vi "Thorlabs Module.vi"(7 "Actions":T3(ring)=enum."Generate Scan Pattern", 8 "error in":errorcluster, 9 "Objective":u16(ring)=1 items=["5X LKM05", "10X LKM10", "20X LKM20", "10X LSM02"], 10 "ROI Parameters":T1={"ROI (mm)"={"X (mm)"=1.0, "Y (mm)"=1.0}, "Shift (mm)"={"Xshift (mm)"=0.0, "Yshift (mm)"=0.0}}, 11 "Scan Parameters":T2={"# Scan"={"#Ascan"=400, "#Bscan"=400}, "# Rpt"={"#ARpt"=1, "#BRpt"=1}, "Aline Rate"=2, "# Extra"={"# ARpt_extra"=5, "#Brtn_extra"=60}} {"Aline Rate" items=["76 KHz", "146 KHz", "76 KHz", "28 KHz", "10 KHz"]}) -> (0 "error out":errorcluster, 2 "Data Out":sgl[][](array[numeric]), 3 "Raw Data Out":u16[][](array[numeric]), 4 "#Blines":dbl)   [LabVIEW 2018]
uses:
  Hardware Mfg/Thorlabs OCT/SpectralRadar/LabVIEW/2012/user.lib/SpectralRadar.llb/Processing Flag Selection.ctl
  Hardware Mfg/Thorlabs OCT/SpectralRadar/LabVIEW/2012/user.lib/SpectralRadar.llb/Probe Parameter Int Selection.ctl
  Hardware Mfg/Thorlabs OCT/SpectralRadar/LabVIEW/2012/user.lib/SpectralRadar.llb/Scan Pattern.lvclass
  Hardware Mfg/Thorlabs OCT/SpectralRadar/LabVIEW/2012/user.lib/SpectralRadar.llb/set Spectrum Output.vi
  Hardware Mfg/Thorlabs OCT/SpectralRadar/LabVIEW/2012/user.lib/SpectralRadar.llb/set Scan Output.vi
  Hardware Mfg/Thorlabs OCT/SpectralRadar/LabVIEW/2012/user.lib/SpectralRadar.llb/Data.lvclass
  Hardware Mfg/Thorlabs OCT/SpectralRadar/LabVIEW/2012/user.lib/SpectralRadar.llb/Raw Data.lvclass
  Hardware Mfg/Thorlabs OCT/SpectralRadar/LabVIEW/2012/user.lib/SpectralRadar.llb/Processing.lvclass
  Hardware Mfg/Thorlabs OCT/SpectralRadar/LabVIEW/2012/user.lib/SpectralRadar.llb/Probe.lvclass
  Hardware Mfg/Thorlabs OCT/SpectralRadar/LabVIEW/2012/user.lib/SpectralRadar.llb/OCT Device.lvclass
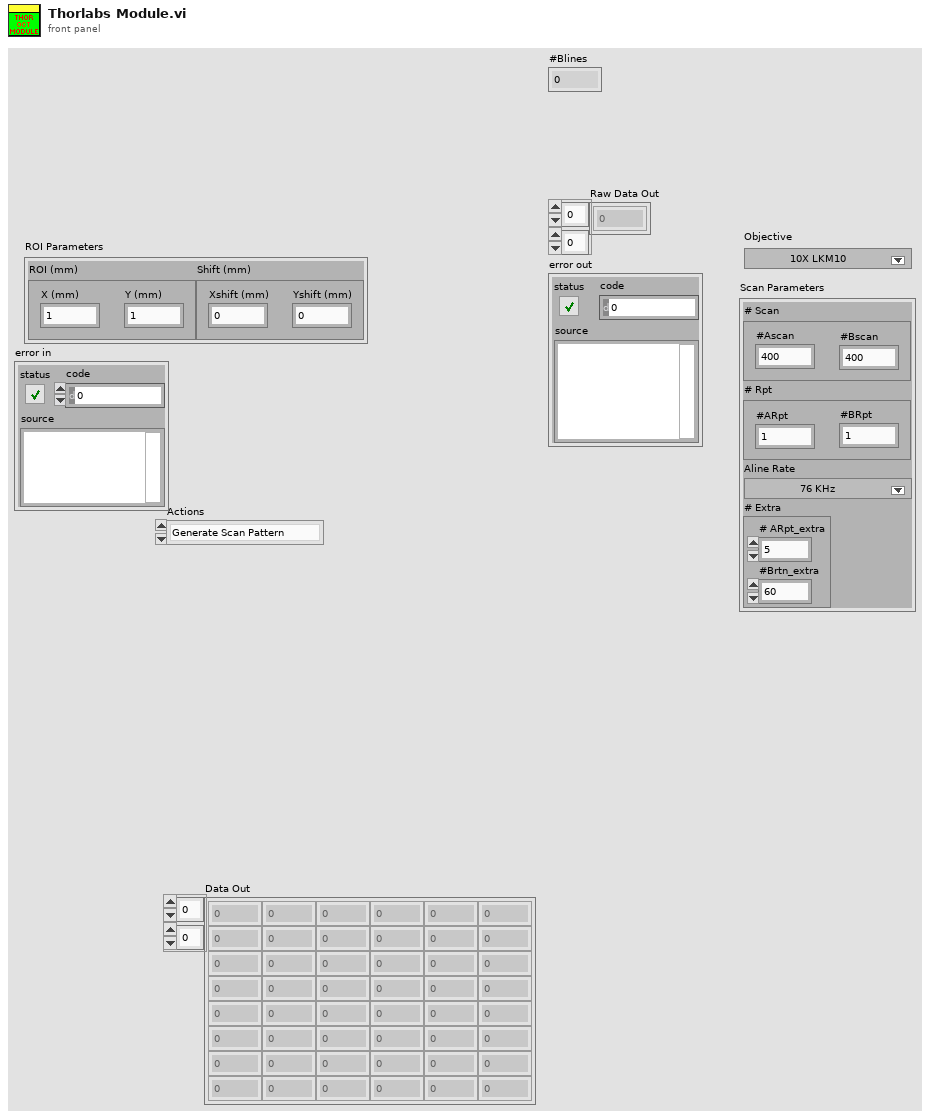
[diagram p1: front panel]
types:
  T1 = cluster{"ROI (mm)":cluster{"X (mm)":dbl, "Y (mm)":dbl}, "Shift (mm)":cluster{"Xshift (mm)":sgl, "Yshift (mm)":sgl}}
  T2 = cluster{"# Scan":cluster{"#Ascan":i32, "#Bscan":i32}, "# Rpt":cluster{"#ARpt":i32, "#BRpt":i32}, "Aline Rate":u16, "# Extra":cluster{"# ARpt_extra":i32, "#Brtn_extra":i32}}
  T3 = enum16{"Init", "Configure", "Configure Data", "Generate Scan Pattern", "Start Acquire Raw", "Start Acquire Data", "Acquire RAW", "Acquire Data", "Stop Acquire", "Uninit"}
  T4 = typedef "Processing.lvclass/Processing Flag Selection.ctl" = enum16{"Use Offset Errors", "Remove DC Spectrum", "Remove Advanced DC Spectrum", "Use Apodization", "Use Scan For Apodization", "Filter Undersampled Signals", "Use Dispersion Compensation", "Use Dechirp", "Use Extended Adjust", "Full Range Output", "Filter DC", "Autocorrelation Compensation", "DEFR", "Only Windowing", "Remove Fixed Pattern"}
  T5 = enum16{"FreeRunning", "TrigBoard_ExternalStart", "External_AScan"}
  T6 = typedef "Probe.lvclass/Probe Parameter Int Selection.ctl" = enum16{"Apodization Cycles", "Oversampling", "White Balance Auto", "Oversampling Slow Axis"}
  T7 = enum16{"Asynchronous Continuous", "Asynchronous Finite", "Synchronous"}
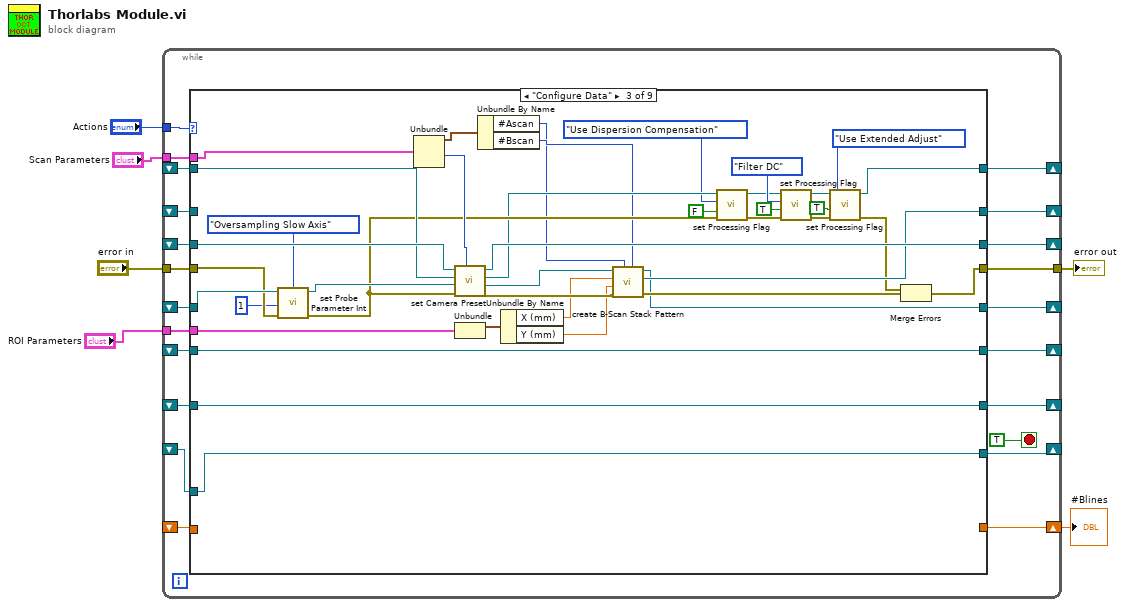
[diagram p0: block diagram]
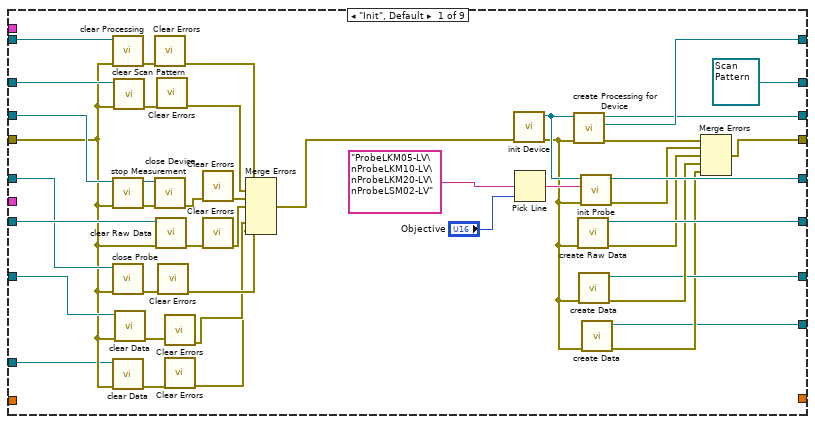
[diagram p2: hidden frame]
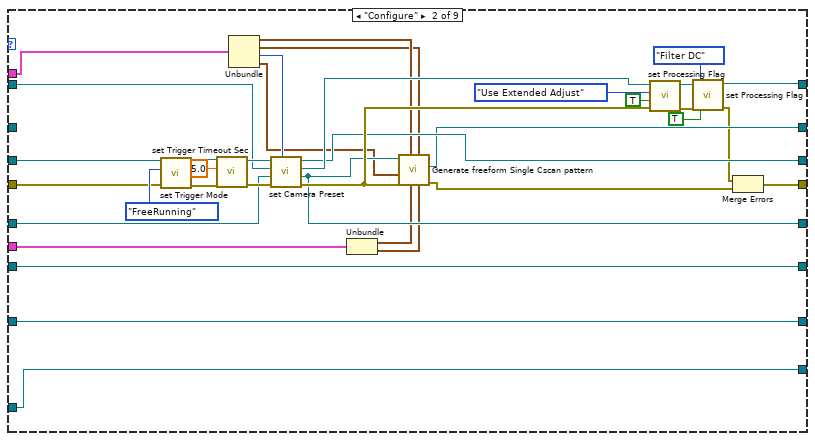
[diagram p3: hidden frame]
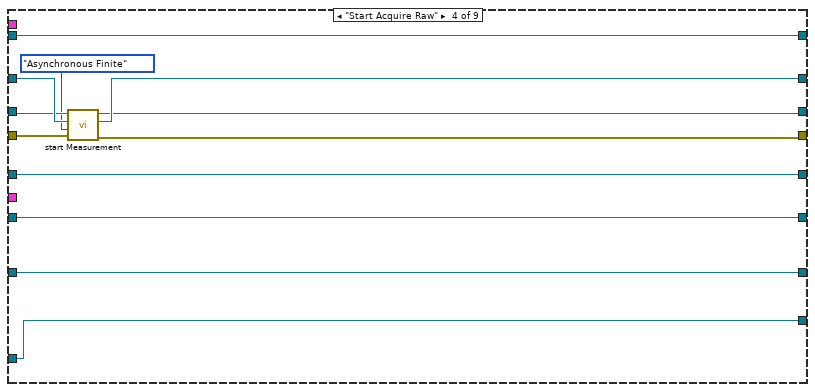
[diagram p4: hidden frame]
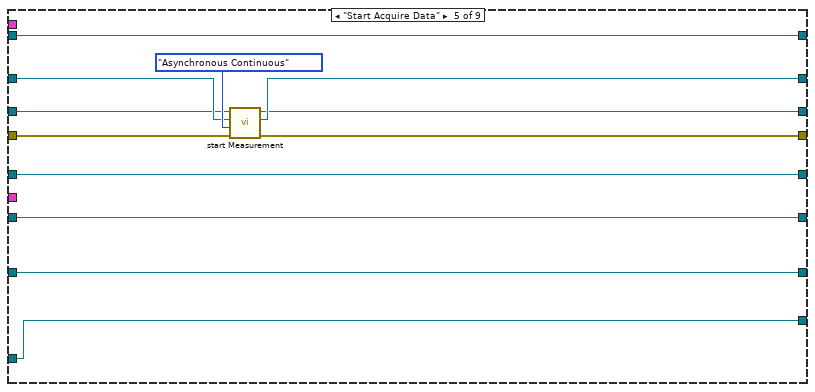
[diagram p5: hidden frame]
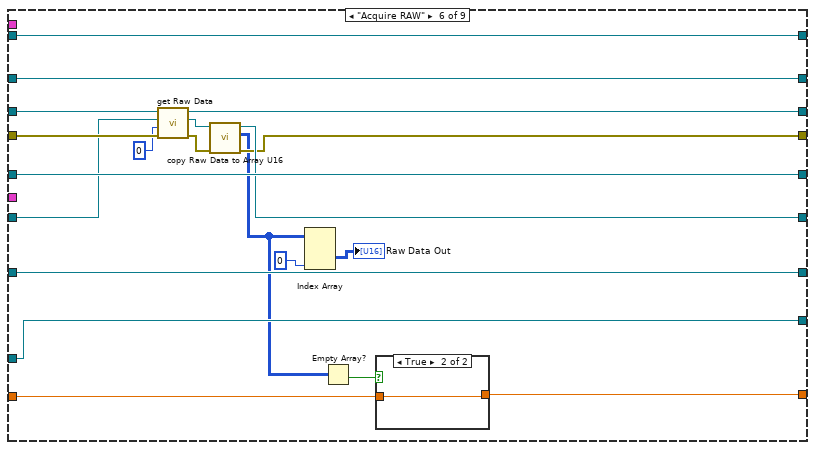
[diagram p6: hidden frame]
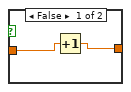
[diagram p7: hidden frame]
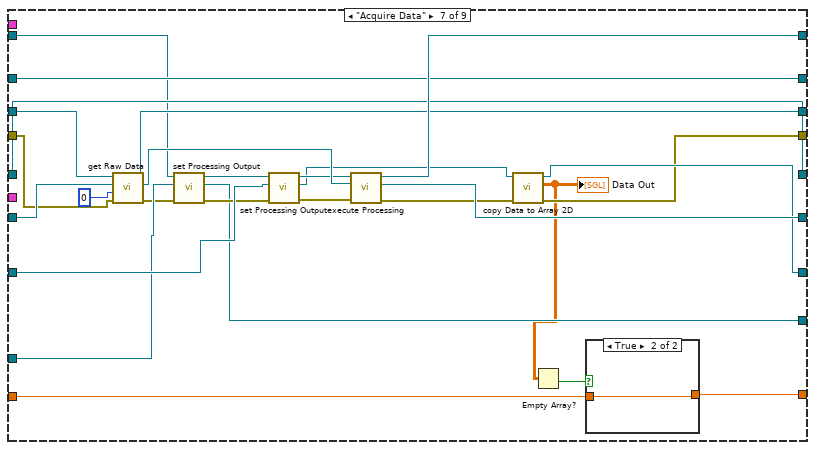
[diagram p8: hidden frame]
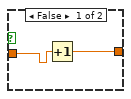
[diagram p9: hidden frame]
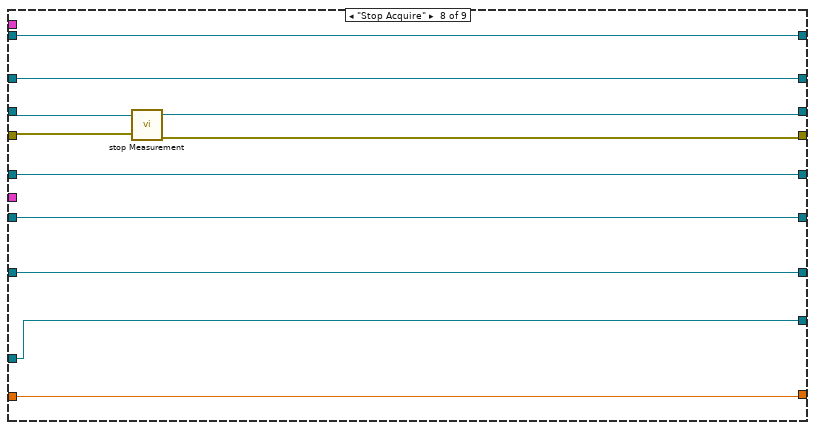
[diagram p10: hidden frame]
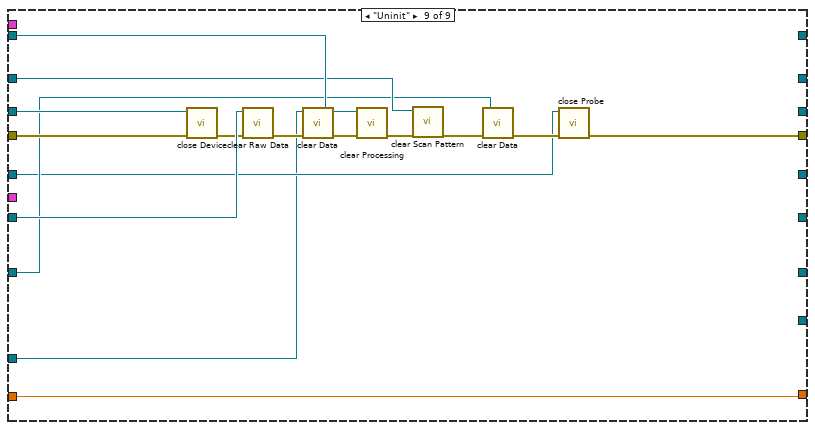
[diagram p11: hidden frame]
diagram:
  n1 = while {
    tunnel: "Actions" -> [w28]
    shift-right: [w26] -> _
    shift-left: _ -> [w22]
    shift-right: [w23] -> _
    shift-left: _ -> [w21]
    shift-right: [w20] -> _
    shift-left: _ -> [w19]
    shift-right: [w18] -> _
    shift-left: _ -> [w17]
    shift-right: [w16] -> _
    shift-left: _ -> [w15]
    tunnel: "error in" -> [w24]
    tunnel: [w25] -> w5
    shift-right: [w14] -> _
    shift-left: _ -> [w13]
    shift-right: [w12] -> _
    shift-left: _ -> [w11]
    tunnel: "Scan Parameters" -> [w10]
    tunnel: "ROI Parameters" -> [w9]
    shift-right: [w8] -> w1
    shift-left: _ -> [w7]
    stop <- TRUE stop-if-true
    n2 = case shown="\"Configure Data\"" w28 {
      tunnel: [w58 w94 w143 w154 w165 w185 w213 w232 _] -> w26
      tunnel: [w64 w106 w132 w158 w169 w180 w199 w234 w241] -> w25
      tunnel: w24 -> [w33 w84 w140 w159 w170 w189 w212 w235 w245]
      tunnel: [w66 w95 w127 w152 w163 w190 w215 w229 _] -> w23
      tunnel: w22 -> [w55 w83 w144 w155 w166 w187 w220 w233 w249]
      tunnel: w21 -> [w52 w78 w142 w152 w163 w190 w215 w229 w240]
      tunnel: [w60 w74 w111 w153 w164 w191 w217 w230 _] -> w20
      tunnel: w19 -> [w50 w85 w137 w153 w164 w191 w209 w230 w248]
      tunnel: [w67 w97 w130 w151 w162 w181 w214 w228 _] -> w18
      tunnel: w17 -> [w53 w97 w130 w151 w162 w186 w221 w228 w251]
      tunnel: [refnum<class "Scan Pattern.lvclass"> refnum ("Scan Pattern") w93 w131 w156 w167 w184 w216 w231 _] -> w16
      tunnel: w15 -> [w51 _ _ w157 w168 w184 w216 w231 w246]
      tunnel: [w45 w82 w129 w149 w161 w177 w202 w227 _] -> w14
      tunnel: w13 -> [w43 w82 w129 w149 w161 w177 w211 w227 w244]
      tunnel: [w34 w81 w128 w148 w160 w176 w201 w226 _] -> w12
      tunnel: w11 -> [w30 w81 w128 w148 w160 w176 w210 w226 w237]
      tunnel: w10 -> [_ w80 w126 _ _ _ _ _ _]
      tunnel: w9 -> [_ w79 w125 _ _ _ _ _ _]
      tunnel: w7 -> [_ _ _ _ _ w173 w196 w225 w236]
      tunnel: [_ _ _ _ _ w172 w195 w225 w236] -> w8
      frame "Init", Default {
        n3 = call "clear Processing.vi"("error in (no error)"=w33, "Processing"=w50) -> ("error out"=w49:errorcluster)  [unwired: 5 in]
        n4 = call "stop Measurement.vi"("error in (no error)"=w33, "OCTDevice"=w55) -> ("error out"=w57:errorcluster, "OCTDevice"=w56:refnum<class "OCT Device.lvclass">)  [unwired: 4 in]
        n5 = call "close Probe.vi"("error in (no error)"=w33, "GalvoControl"=w52) -> ("error out"=w48:errorcluster)  [unwired: 5 in]
        n6 = call "clear Data.vi"("error in (no error)"=w33, "Data"=w30) -> ("error out"=w32:errorcluster)  [unwired: 5 in]
        n7 = call "clear Scan Pattern.vi"("error in (no error)"=w33, "Scan Pattern in"=w51) -> ("error out"=w47:errorcluster)  [unwired: 5 in]
        n8 = call "clear Data.vi"("error in (no error)"=w33, "Data"=w43) -> ("error out"=w44:errorcluster)  [unwired: 5 in]
        n9 = call <vilib>:"Clear Errors.vi"("error in (no error)"=w49) -> ("error out"=w42:errorcluster)  [unwired: 5 in, 1 out]
        n10 = call "close Device.vi"("error in (no error)"=w57, "OCTDevice"=w56) -> ("error out"=w69:errorcluster)  [unwired: 5 in]
        n11 = call "clear Raw Data.vi"("error in (no error)"=w33, "Raw Data"=w53) -> ("error out"=w68:errorcluster)  [unwired: 5 in]
        n12 = call <vilib>:"Clear Errors.vi"("error in (no error)"=w47) -> ("error out"=w41:errorcluster)  [unwired: 5 in, 1 out]
        n13 = call <vilib>:"Clear Errors.vi"("error in (no error)"=w48) -> ("error out"=w38:errorcluster)  [unwired: 5 in, 1 out]
        n14 = call <vilib>:"Clear Errors.vi"("error in (no error)"=w44) -> ("error out"=w37:errorcluster)  [unwired: 5 in, 1 out]
        n15 = call <vilib>:"Clear Errors.vi"("error in (no error)"=w32) -> ("error out"=w31:errorcluster)  [unwired: 5 in, 1 out]
        n16 = call <vilib>:"Clear Errors.vi"("error in (no error)"=w69) -> ("error out"=w40:errorcluster)  [unwired: 5 in, 1 out]
        n17 = call <vilib>:"Clear Errors.vi"("error in (no error)"=w68) -> ("error out"=w39:errorcluster)  [unwired: 5 in, 1 out]
        n18 = Merge Errors(w42, w41, w40, w39, w38, w37, w31) -> (w35:errorcluster)
        n19 = call "init Device.vi"("error in (no error)"=w35) -> ("error out"=w29:errorcluster, "OCTDevice"=w61:refnum<class "OCT Device.lvclass">)  [unwired: 5 in]
        n20 = Pick Line(multi-line string="ProbeLKM05-LV\nProbeLKM10-LV\nProbeLKM20-LV\nProbeLSM02-LV" ("string (\"\")"), line index="Objective") -> (output string=w65:string)  [unwired: 1 in]
        n21 = call "create Processing for Device.vi"("error in (no error)"=w29, "OCTDevice"=w61) -> ("error out"=w59:errorcluster, "Processing"=w60:refnum<class "Processing.lvclass">, "OCTDevice"=w58:refnum<class "OCT Device.lvclass">)  [unwired: 3 in]
        n22 = call "create Raw Data.vi"("error in (no error)"=w29) -> ("error out"=w62:errorcluster, "Raw Data"=w67:refnum<class "Raw Data.lvclass">)  [unwired: 5 in]
        n23 = call "create Data.vi"("error in (no error)"=w29) -> ("error out"=w46:errorcluster, "Data"=w45:refnum<class "Data.lvclass">)  [unwired: 5 in]
        n24 = call "init Probe.vi"("error in (no error)"=w29, "Probe"=w65, "OCT Device"=w61) -> ("error out"=w63:errorcluster, "GalvoControl"=w66:refnum<class "Probe.lvclass">)  [unwired: 3 in]
        n25 = call "create Data.vi"("error in (no error)"=w29) -> ("error out"=w36:errorcluster, "Data"=w34:refnum<class "Data.lvclass">)  [unwired: 5 in]
        n26 = Merge Errors(w59, w63, w62, w46, w36) -> (w64:errorcluster)
      }
      frame "Configure" {
        n27 = call "set Trigger Mode.vi"("error in (no error)"=w84, "Trigger Type"=T5."FreeRunning", "OCTDevice in"=w83) -> ("error out"=w105:errorcluster, "OCTDevice out"=w107:refnum<class "OCT Device.lvclass">)  [unwired: 3 in]
        n28 = call "set Trigger Timeout Sec.vi"("error in (no error)"=w105, "Trigger Timeout"=5.0, "OCTDevice in"=w107) -> ("error out"=w99:errorcluster, "OCTDevice out"=w98:refnum<class "OCT Device.lvclass">)  [unwired: 3 in]
        n29 = Unbundle(w80) -> ("# Scan"=w90:cluster{"#Ascan":i32, "#Bscan":i32}, "# Rpt"=w89:cluster{"#ARpt":i32, "#BRpt":i32}, "Aline Rate"=w91:u16, "# Extra"=w86:cluster{"# ARpt_extra":i32, "#Brtn_extra":i32})
        n30 = call "set Camera Preset.vi"("Numeric"=w91, "error in (no error)"=w99, "Probe"=w78, "Processing"=w85, "OCTDevice"=w98) -> ("error out"=w96:errorcluster, "Probe 2"=w95:refnum<class "Probe.lvclass">, "Processing"=w100:refnum<class "Processing.lvclass">, "OCTDevice out"=w94:refnum<class "OCT Device.lvclass">)  [unwired: 1 in]
        n31 = Unbundle(w79) -> ("ROI (mm)"=w88:cluster{"X (mm)":dbl, "Y (mm)":dbl}, "Shift (mm)"=w87:cluster{"Xshift (mm)":sgl, "Yshift (mm)":sgl})
        n32 = call "Generate freeform Single Cscan pattern.vi"("Shift (mm)"=w87, "# Rpt"=w89, "ROI (mm)"=w88, "# Scan"=w90, "error in (no error)"=w96, "# Extra"=w86, "Probe"=w95) -> ("error out"=w92:errorcluster, "Scan Pattern"=w93:refnum<class "Scan Pattern.lvclass">)  [unwired: 1 in, 2 out]
        n33 = call "set Processing Flag.vi"("error in (no error)"=w96, "Flag"=TRUE, "Processing Flag Selection"=Processing_Flag_Selection."Use Extended Adjust", "Processing"=w100) -> ("error out"=w77:errorcluster, "Processing"=w75:refnum<class "Processing.lvclass">)  [unwired: 2 in]
        n34 = call "set Processing Flag.vi"("error in (no error)"=w77, "Flag"=TRUE, "Processing Flag Selection"=Processing_Flag_Selection."Filter DC", "Processing"=w75) -> ("error out"=w76:errorcluster, "Processing"=w74:refnum<class "Processing.lvclass">)  [unwired: 2 in]
        n35 = Merge Errors(w76, w92) -> (w106:errorcluster)
      }
      frame "Configure Data" {
        n36 = call "set Probe Parameter Int.vi"("error in (no error)"=w140, "Value"=1, "Probe Parameter Int"=Probe_Parameter_Int_Selection."Oversampling Slow Axis", "GalvoControl"=w142) -> ("error out"=w124:errorcluster, "GalvoControl"=w141:refnum<class "Probe.lvclass">)  [unwired: 2 in]
        n37 = Unbundle(w126) -> ("# Scan"=w134:cluster{"#Ascan":i32, "#Bscan":i32}, "Aline Rate"=w147:u16)  [unwired: 2 out]
        n38 = call "set Camera Preset.vi"("Numeric"=w147, "error in (no error)"=w124, "Probe"=w141, "Processing"=w137, "OCTDevice"=w144) -> ("error out"=w136:errorcluster, "Probe 2"=w135:refnum<class "Probe.lvclass">, "Processing"=w118:refnum<class "Processing.lvclass">, "OCTDevice out"=w143:refnum<class "OCT Device.lvclass">)  [unwired: 1 in]
        n39 = Unbundle(w125) -> ("ROI (mm)"=w145:cluster{"X (mm)":dbl, "Y (mm)":dbl})  [unwired: 1 out]
        n40 = Unbundle By Name(w134) -> ("#Ascan"=w108:i32, "#Bscan"=w109:i32)
        n41 = Unbundle By Name(w145) -> ("X (mm)"=w123:dbl, "Y (mm)"=w122:dbl)
        n42 = call "create B-Scan Stack Pattern.vi"("Size Y"=w109, "Size X"=w108, "error in (no error)"=w136, "Range Y"=w122, "Range X"=w123, "Probe"=w135) -> ("error out"=w133:errorcluster, "Scan Pattern"=w131:refnum<class "Scan Pattern.lvclass">, "Probe"=w127:refnum<class "Probe.lvclass">)  [unwired: 1 in]
        n43 = call "set Processing Flag.vi"("error in (no error)"=w124, "Flag"=FALSE, "Processing Flag Selection"=Processing_Flag_Selection."Use Dispersion Compensation", "Processing"=w118) -> ("error out"=w119:errorcluster, "Processing"=w117:refnum<class "Processing.lvclass">)  [unwired: 2 in]
        n44 = call "set Processing Flag.vi"("error in (no error)"=w119, "Flag"=TRUE, "Processing Flag Selection"=Processing_Flag_Selection."Filter DC", "Processing"=w117) -> ("error out"=w146:errorcluster, "Processing"=w112:refnum<class "Processing.lvclass">)  [unwired: 2 in]
        n45 = call "set Processing Flag.vi"("error in (no error)"=w146, "Flag"=TRUE, "Processing Flag Selection"=Processing_Flag_Selection."Use Extended Adjust", "Processing"=w112) -> ("error out"=w114:errorcluster, "Processing"=w111:refnum<class "Processing.lvclass">)  [unwired: 2 in]
        n46 = Merge Errors(w114, w133) -> (w132:errorcluster)
      }
      frame "Start Acquire Raw" {
        n47 = call "start Measurement.vi"("error in (no error)"=w159, "Acquisition Type"=T7."Asynchronous Finite", "Scan Pattern"=w157, "OCTDevice"=w155) -> ("error out"=w158:errorcluster, "Scan Pattern"=w156:refnum<class "Scan Pattern.lvclass">, "OCTDevice"=w154:refnum<class "OCT Device.lvclass">)  [unwired: 1 in]
      }
      frame "Start Acquire Data" {
        n48 = call "start Measurement.vi"("error in (no error)"=w170, "Acquisition Type"=T7."Asynchronous Continuous", "Scan Pattern"=w168, "OCTDevice"=w166) -> ("error out"=w169:errorcluster, "Scan Pattern"=w167:refnum<class "Scan Pattern.lvclass">, "OCTDevice"=w165:refnum<class "OCT Device.lvclass">)  [unwired: 1 in]
      }
      frame "Acquire RAW" {
        n49 = call "get Raw Data.vi"("error in (no error)"=w189, "Camera Index"=0, "RawData in"=w186, "OCTDevice in"=w187) -> ("error out"=w183:errorcluster, "RawData out"=w182:refnum<class "Raw Data.lvclass">, "OCTDevice out"=w185:refnum<class "OCT Device.lvclass">)  [unwired: 1 in]
        n50 = call "copy Raw Data to Array U16.vi"("error in (no error)"=w183, "Data in"=w182) -> ("error out"=w180:errorcluster, "Data Content"=w175:u16[][][], "Data out"=w181:refnum<class "Raw Data.lvclass">)  [unwired: 3 in]
        n51 = Index Array(array=w175, index (dim 2)=0 ("index (page)")) -> (element=→"Raw Data Out":u16[][])  [unwired: 2 in]
        n52 = Empty Array?(array=w175) -> (empty?=w174:bool)
        n53 = case shown="True" w174 {
          tunnel: w173 -> [w193 w194]
          tunnel: [w192 w194] -> w172
          frame False {
            n54 = Increment(x=w193) -> (x+1=w192:dbl)
          }
          frame True {
          }
        }
      }
      frame "Acquire Data" {
        n55 = call "get Raw Data.vi"("error in (no error)"=w212, "Camera Index"=0, "RawData in"=w221, "OCTDevice in"=w220) -> ("error out"=w208:errorcluster, "RawData out"=w218:refnum<class "Raw Data.lvclass">, "OCTDevice out"=w213:refnum<class "OCT Device.lvclass">)  [unwired: 1 in]
        n56 = call-poly "set Processing Output.vi"("error in (no error)"=w208, "Data"=w210, "Processing"=w209) -> ("error out"=w207:errorcluster, "Data"=w201:refnum<class "Data.lvclass">, "Processing"=w205:refnum<class "Processing.lvclass">)  [unwired: 2 in]
        n57 = call-poly "set Processing Output.vi"("error in (no error)"=w207, "Data"=w211, "Processing"=w205) -> ("error out"=w219:errorcluster, "Data"=w203:refnum<class "Data.lvclass">, "Processing"=w204:refnum<class "Processing.lvclass">)  [unwired: 2 in]
        n58 = call "execute Processing.vi"("error in (no error)"=w219, "Raw Data"=w218, "Processing"=w204) -> ("error out"=w200:errorcluster, "Raw Data"=w214:refnum<class "Raw Data.lvclass">, "Processing"=w217:refnum<class "Processing.lvclass">)  [unwired: 2 in]
        n59 = call "copy Data to Array 2D.vi"("error in (no error)"=w200, "Data in"=w203) -> ("error out"=w199:errorcluster, "Data Content"=w197:sgl[][], "Data out"=w202:refnum<class "Data.lvclass">)  [unwired: 3 in]
        "Data Out" <- w197
        n60 = Empty Array?(array=w197) -> (empty?=w198:bool)
        n61 = case shown="True" w198 {
          tunnel: w196 -> [w223 w224]
          tunnel: [w222 w224] -> w195
          frame False {
            n62 = Increment(x=w223) -> (x+1=w222:dbl)
          }
          frame True {
          }
        }
      }
      frame "Stop Acquire" {
        n63 = call "stop Measurement.vi"("error in (no error)"=w235, "OCTDevice"=w233) -> ("error out"=w234:errorcluster, "OCTDevice"=w232:refnum<class "OCT Device.lvclass">)  [unwired: 4 in]
      }
      frame "Uninit" {
        n64 = call "close Device.vi"("error in (no error)"=w245, "OCTDevice"=w249) -> ("error out"=w250:errorcluster)  [unwired: 5 in]
        n65 = call "clear Raw Data.vi"("error in (no error)"=w250, "Raw Data"=w251) -> ("error out"=w239:errorcluster)  [unwired: 5 in]
        n66 = call "clear Data.vi"("error in (no error)"=w239, "Data"=w237) -> ("error out"=w238:errorcluster)  [unwired: 5 in]
        n67 = call "clear Processing.vi"("error in (no error)"=w238, "Processing"=w248) -> ("error out"=w247:errorcluster)  [unwired: 5 in]
        n68 = call "clear Scan Pattern.vi"("error in (no error)"=w247, "Scan Pattern in"=w246) -> ("error out"=w243:errorcluster)  [unwired: 5 in]
        n69 = call "clear Data.vi"("error in (no error)"=w243, "Data"=w244) -> ("error out"=w242:errorcluster)  [unwired: 5 in]
        n70 = call "close Probe.vi"("error in (no error)"=w242, "GalvoControl"=w240) -> ("error out"=w241:errorcluster)  [unwired: 5 in]
      }
    }
  }
  "error out" <- w5
  "#Blines" <- w1
